vi "uintHeapSort.vi"(8 "Error in (no error)":errorcluster, 11 "Uint array in":refnum<class "UintClass.lvclass">[](array[class])) -> (0 "Error out":errorcluster, 1 "Timing":u32, 3 "Sorted uint array":refnum<class "UintClass.lvclass">[](array[class]))   [LabVIEW 2011, in "UintClass.lvclass"]
uses:
  UintClass.lvclass
  uintGreater.vi
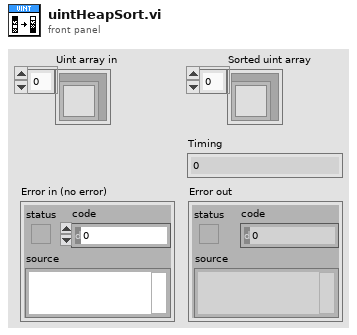
[diagram p1: front panel]
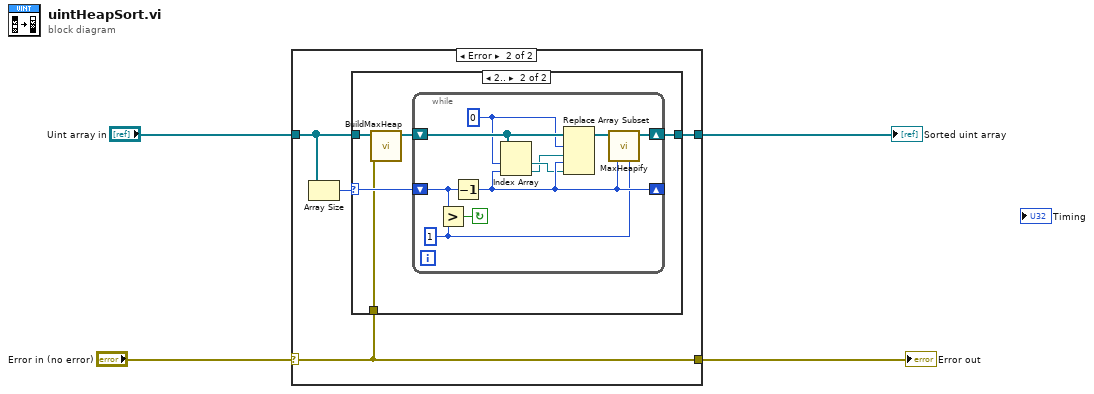
[diagram p0: block diagram]
diagram:
  n1 = case shown="Error" "Error in (no error)" {
    selector: "Error in (no error)" -> [w5 w6]
    tunnel: [w5 w6] -> w3
    tunnel: "Uint array in" -> [_ w8]
    tunnel: [_ w7] -> w1
    frame No Error {
    }
    frame Error {
      n2 = Array Size(array=w8) -> (size(s)=w9:i32)
      n3 = case shown="2.." w9 {
        selector: w9 -> [_ w12]
        tunnel: [w10 w14] -> w7
        tunnel: w8 -> [w10 w13]
        tunnel: w6 -> [_ w11]
        frame ..1 {
        }
        frame 2.. {
          n4 = call "BuildMaxHeap.vi"("Error in (no error)"=w11, "Heap in"=w13) -> ("Heap out"=w15:refnum<class "UintClass.lvclass">[])  [unwired: 8 in, 1 out]
          n5 = while {
            shift-right: [w19] -> _
            shift-left: w12 -> [w24]
            shift-right: [w22] -> w14
            shift-left: w15 -> [w21]
            stop <- w25 continue-if-true
            w20 = 0 ("index")
            w16 = 1 ("y")
            n6 = Greater?(x=w24, y=w16) -> (0:w25:bool)
            n7 = Decrement(x=w24) -> (x-1=w19:i32)
            n8 = Index Array(array=w21, index #1=w20, index #2=w19) -> (element #1=w18:refnum<class "UintClass.lvclass">, element #2=w17:refnum<class "UintClass.lvclass">)
            n9 = Replace Array Subset(array=w21, new element #1=w17, index #1=w20, new element #2=w18, index #2=w19) -> (w23:refnum<class "UintClass.lvclass">[])
            n10 = call "MaxHeapify.vi"("Length"=w19, "i"=w16, "Heap in"=w23) -> ("Heap out"=w22:refnum<class "UintClass.lvclass">[])  [unwired: 7 in, 1 out]
          }
        }
      }
    }
  }
  "Sorted uint array" <- w1
  "Error out" <- w3
